vi "Read Transfer.vi"(8 "error in (no error)":errorcluster, 10 "Transfer ID":string, 11 "dsf refnum":T1) -> (0 "error out":errorcluster, 1 "value":T2, 3 "dsf refnum out":T1, 4 "found?":bool)   [LabVIEW 2017, in "DSF Core.lvlib"]
doc: "Reads a value associated with a key in a specified section from the configuration data identified by <B>dsf refnum</B>. If the key does not exist, the VI returns the default value. This VI supports multibyte characters in strings. Wire data to the <B>default value</B> input to determine the polymorphic instance to use or manually select the instance."
uses:
  DSF Core.lvlib
  Controls/DSF Transfer Info.ctl
  Controls/DSF Byte Order.ctl
  Controls/DSF Config Data RefNum.ctl
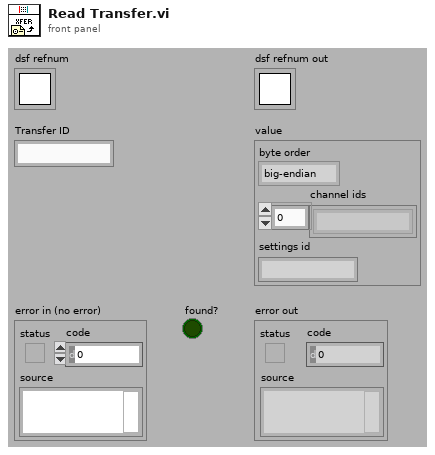
[diagram p1: front panel]
types:
  T1 = typedef "DSF Core.lvlib/DSF Config Data RefNum.ctl" = refnum<k1>
  T2 = typedef "DSF Core.lvlib/DSF Transfer Info.ctl" = cluster{"byte order":T3, "channel ids":string[], "settings id":string}
  T3 = typedef "DSF Core.lvlib/DSF Byte Order.ctl" = enum8{"big-endian", "little-endian"}
  T4 = typedef "DSF Core.lvlib/DSF Configuration Reference.ctl" = refnum<data-value>
  T5 = typedef "DSF Core.lvlib/Internal.DSF Configuration.ctl" = cluster{"dsfversion":T6, "version":T6, "plugins":T7[], "groups":T10[], "transfers":T12[], "channels":T14[], "settings":T16[]}
  T6 = typedef "DSF Core.lvlib/DSF Version Info.ctl" = cluster{"major":u32, "minor":u32, "fix":u32, "build":string}
  T7 = typedef "DSF Core.lvlib/Internal.DSF Plugin with ID.ctl" = cluster{"id":string, "values":T8}
  T8 = typedef "DSF Core.lvlib/Internal.DSF Plugin Info.ctl" = cluster{"type":string, "timing":T9, "group ids":string[], "settings id":string}
  T9 = typedef "DSF Core.lvlib/DSF Timing Info.ctl" = cluster{"priority":u64, "decimation":u64, "offset":u64}
  T10 = typedef "DSF Core.lvlib/Internal.DSF Group with ID.ctl" = cluster{"id":string, "values":T11}
  T11 = typedef "DSF Core.lvlib/Internal.DSF Group Info.ctl" = cluster{"direction":i32, "timing":T9, "transfer ids":string[], "settings id":string}
  T12 = typedef "DSF Core.lvlib/Internal.DSF Transfer with ID.ctl" = cluster{"id":string, "values":T13}
  T13 = typedef "DSF Core.lvlib/Internal.DSF Transfer Info.ctl" = cluster{"byte order":i32, "channel ids":string[], "settings id":string}
  T14 = typedef "DSF Core.lvlib/Internal.DSF Channel with ID.ctl" = cluster{"id":string, "values":T15}
  T15 = typedef "DSF Core.lvlib/Internal.DSF Channel Info.ctl" = cluster{"count":u64, "buffer offset":u64, "data type":i32, "settings id":string}
  T16 = typedef "DSF Core.lvlib/Internal.DSF Settings with ID.ctl" = cluster{"id":string, "values":T17}
  T17 = typedef "DSF Core.lvlib/Internal.DSF Settings Info.ctl" = cluster{"key":string, "value":string}[]
  T18 = cluster{"dsf configuration":T5, "path":path, "dirty":bool}
  T19 = typedef "DSF Core.lvlib/DSF Config Data.ctl" = cluster{"dsf configuration":T5, "path":path, "dirty":bool}
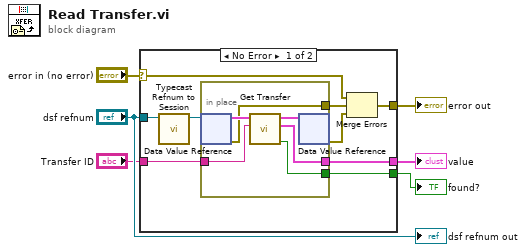
[diagram p0: block diagram]
diagram:
  n1 = case shown="No Error" "error in (no error)" {
    selector: "error in (no error)" -> [w15 w22]
    tunnel: "dsf refnum" -> [w14 _]
    tunnel: [w9 w22] -> w4
    tunnel: "Transfer ID" -> [w13 _]
    tunnel: [w12 _] -> w2
    tunnel: [w11 _] -> w1
    frame No Error {
      n2 = call "Typecast Refnum to Session.vi"("dsf refnum in"=w14) -> ("DSF Configuration Session out"=w10:T4)  [unwired: 10 in]
      n3 = in-place {
        in-place-border: w13 -> [w21]
        in-place-border: [w20] -> w12
        in-place-border: [w19] -> w11
        in-place-border: [w16] -> w8
        n4 = in-place-dvr #1(w10) -> (w18:T18, w16:errorcluster)
        n5 = call "Get Transfer.vi"("id"=w21, "DSF Configuration in"=w18) -> ("exists?"=w19:bool, "info"=w20:T2, "DSF Configuration out"=w17:T19)  [unwired: 6 in, 1 out]
        n6 = in-place-dvr #1(w17) -> (w7:errorcluster)  [unwired: 1 out]
      }
      n7 = Merge Errors(w15, w8, w7) -> (w9:errorcluster)
    }
    frame Error {
    }
  }
  "error out" <- w4
  "found?" <- w1
  "value" <- w2
  "dsf refnum out" <- "dsf refnum"
